vi "Array 2.vi"() -> ()   [LabVIEW 2014]
uses:
  <vilib>/Aledyne-TSXperts/Arduino Compatible Compiler for LabVIEW/addons/Arduino SoftwareSerial Wrapper/Arduino SoftwareSerial Wrapper.lvlib
panel:
  out "Bytes written":u8
  out "Error Out":errorcluster
  in  "Error In":errorcluster
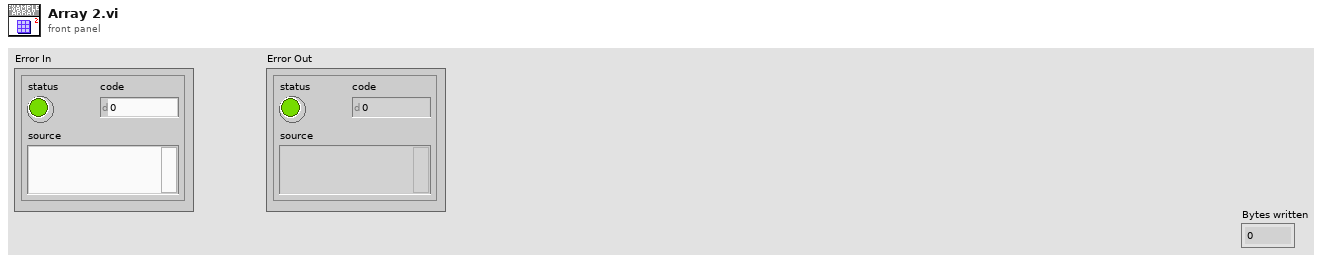
[diagram p1: front panel]
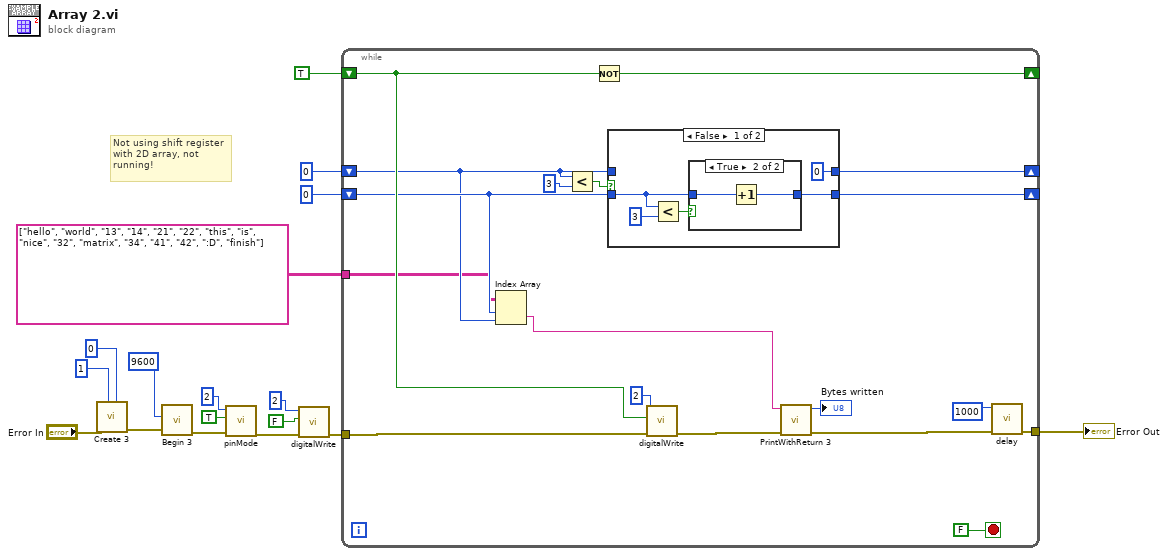
[diagram p0: block diagram]
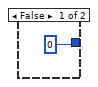
[diagram p2: hidden frame]
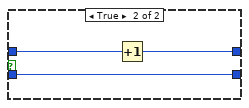
[diagram p3: hidden frame]
diagram:
  # "Not using shift register with 2D array, not running!"
  n1 = call <userlib>:"Create 3.vi"("arduino RX pin"=u8 0, "arduino TX pin"=u8 1, "Error In"="Error In") -> ("Error Out"=w10:errorcluster)  [unwired: 8 in]
  n2 = call <userlib>:"Begin 3.vi"("Error In"=w10, "Baudrate"=u16 9600) -> ("Error Out"=w8:errorcluster)  [unwired: 8 in]
  n3 = call "pinMode.vi"("Error In"=w8, "output?"=TRUE, "pin number"=2) -> ("Error Out"=w3:errorcluster)  [unwired: 8 in]
  n4 = call "digitalWrite.vi"("Error In"=w3, "value"=FALSE, "pin number"=2) -> ("Error Out"=w4:errorcluster)  [unwired: 8 in]
  n5 = while {
    tunnel: [w33] -> w15
    shift-right: [w27] -> _
    shift-left: 0 ("index") -> [w21]
    shift-right: [w32] -> _
    shift-left: TRUE -> [w30]
    tunnel: w4 -> [w31]
    shift-right: [w26] -> _
    shift-left: 0 ("index") -> [w22]
    tunnel: string[][] [["hello", "world", "13", "14"], ["21", "22", "this", "is"], ["nice", "32", "matrix", "34"], ["41", "42", ":D", "finish"]] -> [w19]
    stop <- FALSE stop-if-true
    n6 = Index Array(array=w19, index (row)=w22, index (col)=w21) -> (element=w20:string)
    n7 = Less?(x=w21, y=3) -> (x < y?=w29:bool)
    n8 = Not(x=w30) -> (.not. x?=w32:bool)
    n9 = case shown="False" w29 {
      tunnel: w21 -> [_ w46]
      tunnel: [0 w45] -> w27
      tunnel: w22 -> [w37 w44]
      tunnel: [w36 w44] -> w26
      frame False {
        n10 = Less?(x=w37, y=3) -> (x < y?=w38:bool)
        n11 = case shown="True" w38 {
          tunnel: w37 -> [_ w43]
          tunnel: [0 w42] -> w36
          frame False {
          }
          frame True {
            n12 = Increment(x=w43) -> (x+1=w42:i32)
          }
        }
      }
      frame True {
        n13 = Increment(x=w46) -> (x+1=w45:i32)
      }
    }
    n14 = call "digitalWrite.vi"("Error In"=w31, "value"=w30, "pin number"=2) -> ("Error Out"=w23:errorcluster)  [unwired: 8 in]
    n15 = call <userlib>:"PrintWithReturn 3.vi"("Error In"=w23, "String to print"=w20) -> ("Error Out"=w24:errorcluster, "Bytes written"=→"Bytes written":u8)  [unwired: 8 in]
    n16 = call "delay.vi"("Error In"=w24, "time (ms)"=1000) -> ("Error Out"=w33:errorcluster)  [unwired: 9 in]
  }
  "Error Out" <- w15
